vi "solar_misc Delta Time.vi"(4 "error in (no error)":errorcluster, 8 "Previous Time (sec)":dbl format="%#.9f") -> (1 "error out":errorcluster, 5 "Current Time (sec)":dbl format="%#.9f", 7 "Delta (ms)":u32)   [LabVIEW 2018]
doc: "This calculates the delta time. Useful for debuging execution time."
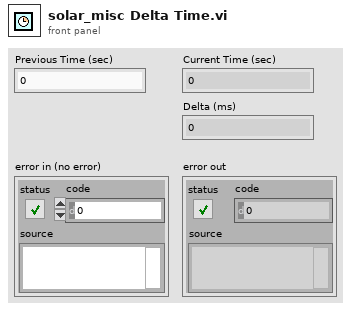
[diagram p1: front panel]
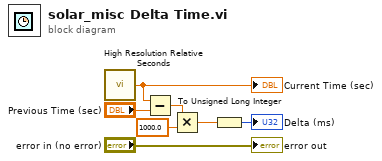
[diagram p0: block diagram]
diagram:
  n1 = call <vilib>:"High Resolution Relative Seconds.vi"() -> ("relative seconds"=w7:dbl)
  "Current Time (sec)" <- w7
  n2 = Subtract(x=w7, y="Previous Time (sec)") -> (x-y=w5:dbl)
  n3 = Multiply(x=w5, y=1000.0) -> (x*y=w3:dbl)
  n4 = To Unsigned Long Integer(number=w3) -> (unsigned 32bit integer=→"Delta (ms)":u32)
  "error out" <- "error in (no error)"
